vi "Load Simple Explorer.vi"(8 "error in (no error)":errorcluster, 10 "Configuration Session":refnum<class "Configuration Session.lvclass">=refnum, 11 "Item Ref in":T2 format="%.0x") -> (0 "error out":errorcluster, 3 "Item Ref out":T2 format="%.0x")   [LabVIEW 2019]
uses:
  <vilib>/NI VeriStand/Custom Device API/Custom Device API.lvlib
  DSF Core.lvlibp/Classes/Configuration/Configuration Session.lvclass
  <vilib>/NI VeriStand/Custom Device API/Get Item Property (String).vi
  <vilib>/NI VeriStand/Custom Device API/Custom Device Item Ref.ctl
  Development Tools/Data Sharing Configuration Explorer/Source/Item Tree/ID to Tree Items/Tree Item Type.ctl
panel:
  in  "Item Type":T1
  out "reference out":refnum<vi>
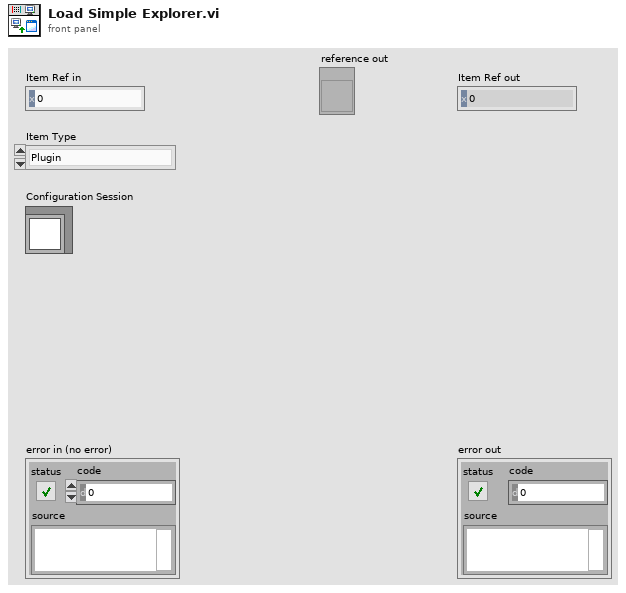
[diagram p1: front panel]
types:
  T1 = typedef "DSF Configuration Utility.lvlib/Tree Item Type.ctl" = enum16{"Plugin", "Group", "Transfer", "Channel", "Setting"}
  T2 = typedef "Custom Device API.lvlib/Custom Device Item Ref.ctl" = u64
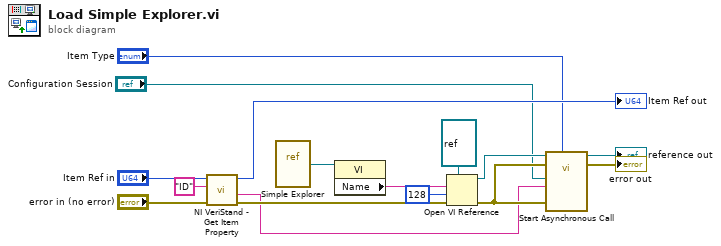
[diagram p0: block diagram]
diagram:
  n1 = call-poly <vilib>:"NI VeriStand - Get Item Property.vi"("error in (no error)"="error in (no error)", "Property Name"="ID", "Item Ref in"="Item Ref in") -> ("error out"=w6:errorcluster, "Value"=w4:string, "Item Ref out"=→"Item Ref out":T2)  [unwired: 5 in, 1 out]
  n2 = vi-ref "Simple Explorer.vi"() -> (w13:refnum<vi>)
  n3 = property class="VI"(reference=w13) -> ("Name"=w12:string)  [unwired: 1 in, 2 out]
  n4 = Open VI Reference(type specifier VI Refnum (for type only)=refnum<vi> refnum, vi path=w12, options=128, error in (no error)=w6) -> (vi reference=w10:refnum<vi>, error out=w14:errorcluster)  [unwired: 2 in]
  n5 = call-by-ref "Start Asynchronous Call"(reference=w10, error in=w14, "Item Type"="Item Type", 8:"error in (no error)"=w14, "Item ID"=w4, "Configuration Session"="Configuration Session") -> (reference out=→"reference out":refnum<vi>, error out=→"error out":errorcluster)  [unwired: 7 in, 1 out]
